vi "MBThinkDynamicTest.vi"() -> ()   [LabVIEW 2013]
doc: "Use this to get a feel for the MB decision maker in \"real\" time, and test it out, try and find bugs.\n\nFeb. 2014, Eric Schneider"
uses:
  Data/TypeDefs/Boat Regimes.ctl
  Data/TypeDefs/Sailing Regimes.ctl
  Data/TypeDefs/Emergency Regimes.ctl
  Data/TypeDefs/Rudder Set Suggestions.ctl
  Data/TypeDefs/Sail Set Suggestions.ctl
  Data/TypeDefs/JibPositionIndicator.ctl
  Data/TypeDefs/MainsailPositionIndicator.ctl
  Utilities/Math/Angles/Angle/Angle.lvclass
panel:
  out "Mainsail\nPosition":T1
  out "Jib\nPosition":T2
  out "Suggested Sail Setpoints":T3 {"MainSailSuggestion" min=0.0 max=1.0; "JibSailSuggestion" min=0.0 max=1.0}
  out "Suggested Rudder Setpoint":T4 min=-1.0 max=1.0 scale=1.0..-1.0
  out "Heartbeat":bool
  in  "Loop period (ms)":u32(knob)=259 scale=0.0..500.0
  out "Last Commanded Boat Regime":T5={"Sailing Regime"=enum."Upwind - Starboard Tack", "Emergency Regimes"=enum."NO EMERGENCY", "Emergency?"=FALSE}
  in  "Trusted Absolute Wind Data (deg)":dbl(knob)
  in  "Robot Heading (deg)":dbl(knob)
  out "Commanded Boat Regime":T5
  in  "Desired Heading (deg)":dbl(knob)
  in  "stop":bool
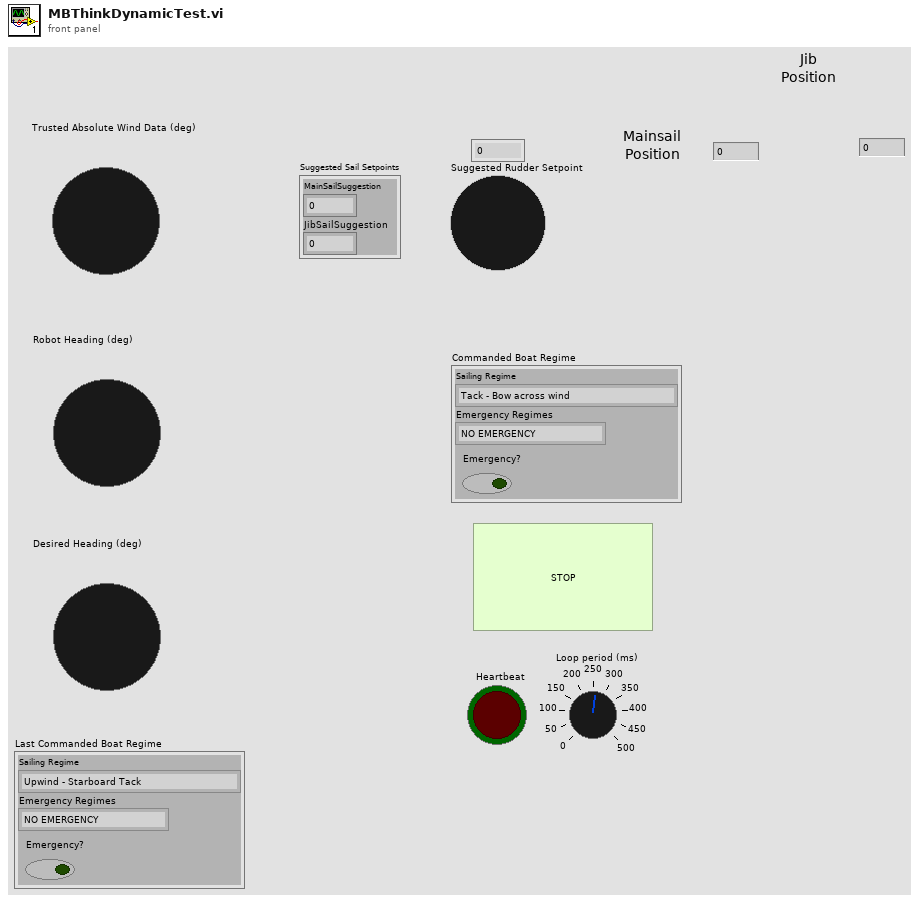
[diagram p1: front panel]
types:
  T1 = typedef "MainsailPositionIndicator.ctl" = dbl
  T2 = typedef "JibPositionIndicator.ctl" = dbl
  T3 = typedef "Sail Set Suggestions.ctl" = cluster{"MainSailSuggestion":dbl, "JibSailSuggestion":dbl}
  T4 = typedef "Rudder Set Suggestions.ctl" = dbl
  T5 = typedef "Boat Regimes.ctl" = cluster{"Sailing Regime":T6, "Emergency Regimes":T7, "Emergency?":bool}
  T6 = typedef "Sailing Regimes.ctl" = enum16{"Tack - Bow across wind", "Upwind - Starboard Tack", "Turn between Upwind/Reach - Starboard Tack", "Reach - Starboard Tack", "Turn between Reach/Run - Starboard Tack", "Run - Starboard Tack", "Jibe - Stern across wind", "Run - Port Tack", "Turn between Reach/Run - Port Tack", "Reach - Port Tack", "Turn between Upwind/Reach - Port Tack", "Upwind - Port Tack"}
  T7 = typedef "Emergency Regimes.ctl" = enum16{"NO EMERGENCY", "No Knockdown", "Obstacle Avoid"}
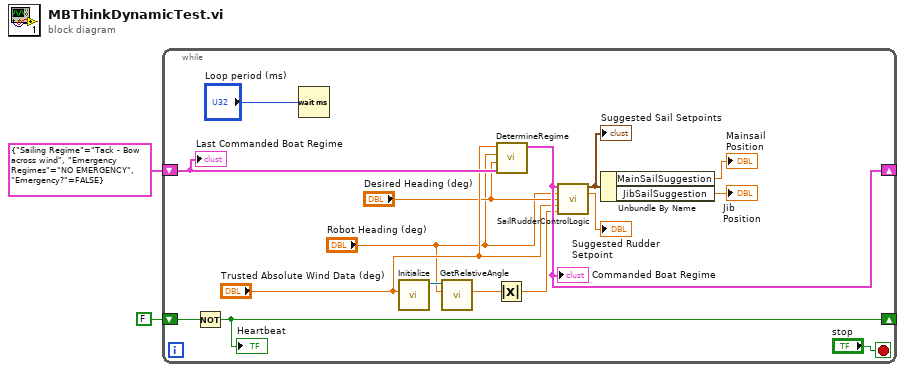
[diagram p0: block diagram]
diagram:
  n1 = while {
    shift-right: [w13] -> _
    shift-left: T5 {"Sailing Regime"=enum."Tack - Bow across wind", "Emergency Regimes"=enum."NO EMERGENCY", "Emergency?"=FALSE} ("Commanded Boat Regime") -> [w17]
    shift-right: [w14] -> _
    shift-left: FALSE -> [w15]
    stop <- "stop" stop-if-true
    n2 = Not(x=w15) -> (.not. x?=w14:bool)
    "Heartbeat" <- w14
    n3 = Wait (ms)(milliseconds to wait="Loop period (ms)") -> ()  [unwired: 1 out]
    n4 = call "Initialize.vi"("Input Angle (Deg.)"="Trusted Absolute Wind Data (deg)") -> ("Angle out"=w11:refnum<class "Angle.lvclass">)  [unwired: 9 in, 1 out]
    n5 = call "GetRelativeAngle.vi"("Boat Heading (Deg.)"="Robot Heading (deg)", "Angle in"=w11) -> ("Relative Angle"=w10:dbl)  [unwired: 8 in, 1 out]
    n6 = Absolute Value(x=w10) -> (abs(x)=w9:dbl)
    n7 = call "DetermineRegime.vi"("Last Commanded Boat Regime"=w17, "Desired Heading (deg)"="Desired Heading (deg)", "Robot Heading (deg)"="Robot Heading (deg)", "Trusted Absolute Wind Data (deg)"="Trusted Absolute Wind Data (deg)") -> ("Commanded Boat Regime"=w13:T5)  [unwired: 7 in]
    "Commanded Boat Regime" <- w13
    n8 = call "SailRudderControlLogic.vi"("Commanded Boat Regime"=w13, "Robot Heading"="Robot Heading (deg)", "DesiredHeading"="Desired Heading (deg)", "AbsoluteWindAngle"="Trusted Absolute Wind Data (deg)", "ApparentWindAngle (0-180)"=w9) -> ("Suggested Sail Setpoints"=w5:T3, "Suggested Rudder Setpoint"=→"Suggested Rudder Setpoint":T4)  [unwired: 9 in]
    "Suggested Sail Setpoints" <- w5
    n9 = Unbundle By Name(w5) -> ("MainSailSuggestion"=→"Mainsail\nPosition":dbl, "JibSailSuggestion"=→"Jib\nPosition":dbl)
    "Last Commanded Boat Regime" <- w17
  }
